vi "WLAN - BCM - PL.vi"(6 "RX ?":bool, 11 "Channel index":i32=1) -> (3 "PL":dbl=17.6)   [LabVIEW 2012]
panel:
  in  "PL_channel Index":dbl[](array[numeric])=[0.0, 17.6, 0.0, 0.0, 0.0, 0.0, 0.0, 17.4, 0.0, 0.0, 0.0, 0.0, 0.0, 17.2, 0.0, 0.0, 0.0, 0.0, 0.0, 0.0, 0.0, 0.0, 0.0, 0.0, 0.0, 0.0, 0.0, 0.0, 0.0, 0.0, 0.0, 0.0, 0.0, 0.0, 0.0, 0.0, 16.5, 0.0, 17.6, 0.0, 0.0, 0.0, 0.0, 0.0, 0.0, 0.0, 17.75, 0.0, 0.0, 0.0, 0.0, 0.0, 16.75, 0.0, 0.0, 0.0, 0.0, 0.0, 0.0, 0.0, 0.0, 0.0, 17.75, 0.0, 16.75, 0.0, 0.0, 0.0, 0.0, 0.0, 0.0, 0.0, 0.0, 0.0, 0.0, 0.0, 0.0, 0.0, 0.0, 0.0, 0.0, 0.0, 0.0, 0.0, 0.0, 0.0, 0.0, 0.0, 0.0, 0.0, 0.0, 0.0, 0.0, 0.0, 0.0, 0.0, 0.0, 0.0, 0.0, 0.0, 16.75, 0.0, 17.9, 0.0, 0.0, 0.0, 0.0, 0.0, 0.0, 0.0, 0.0, 0.0, 0.0, 0.0, 0.0, 0.0, 0.0, 0.0, 0.0, 0.0, 16.75, 0.0, 0.0, 0.0, 0.0, 0.0, 17.9, 0.0, 0.0, 0.0, 0.0, 0.0, 0.0, 0.0, 17.7, 0.0, 0.0, 0.0, 0.0, 0.0, 16.7, 0.0, 0.0, 0.0, 0.0, 0.0, 0.0, 0.0, 0.0, 16.5, 0.0, 17.8, 0.0, 0.0, 0.0, 0.0, 0.0, 16.75, 0.0, 17.9, 0.0, 0.0, 0.0, 0.0, 0.0, 16.75]
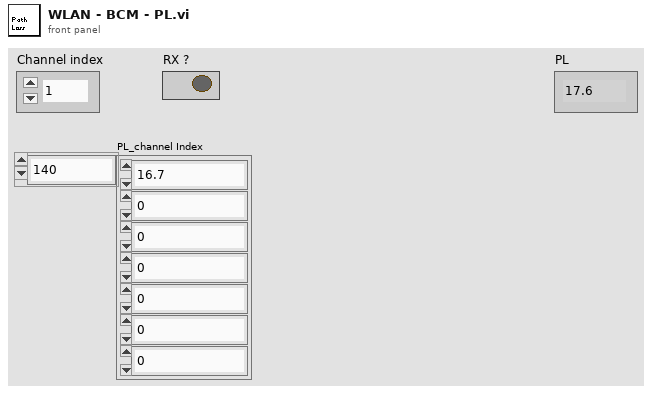
[diagram p1: front panel]
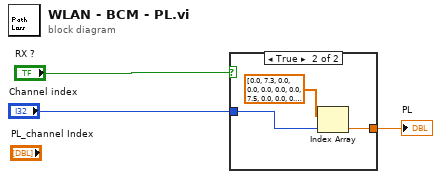
[diagram p0: block diagram]
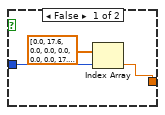
[diagram p2: hidden frame]
diagram:
  n1 = case shown="True" "RX ?" {
    tunnel: [w5 w7] -> w2
    tunnel: "Channel index" -> [w4 w8]
    frame False {
      n2 = Index Array(array=dbl[] [0.0, 17.6, 0.0, 0.0, 0.0, 0.0, 0.0, 17.4, 0.0, 0.0, 0.0, 0.0, 0.0, 17.2, 0.0, 0.0, 0.0, 0.0, 0.0, 0.0, 0.0, 0.0, 0.0, 0.0, 0.0, 0.0, 0.0, 0.0, 0.0, 0.0, 0.0, 0.0, 0.0, 0.0, 0.0, 0.0, 16.5, 0.0, 17.6, 0.0, 0.0, 0.0, 0.0, 0.0, 0.0, 0.0, 17.75, 0.0, 0.0, 0.0, 0.0, 0.0, 16.75, 0.0, 0.0, 0.0, 0.0, 0.0, 0.0, 0.0, 0.0, 0.0, 17.75, 0.0, 16.75, 0.0, 0.0, 0.0, 0.0, 0.0, 0.0, 0.0, 0.0, 0.0, 0.0, 0.0, 0.0, 0.0, 0.0, 0.0, 0.0, 0.0, 0.0, 0.0, 0.0, 0.0, 0.0, 0.0, 0.0, 0.0, 0.0, 0.0, 0.0, 0.0, 0.0, 0.0, 0.0, 0.0, 0.0, 0.0, 16.75, 0.0, 17.9, 0.0, 0.0, 0.0, 0.0, 0.0, 0.0, 0.0, 0.0, 0.0, 0.0, 0.0, 0.0, 0.0, 0.0, 0.0, 0.0, 0.0, 16.75, 0.0, 0.0, 0.0, 0.0, 0.0, 17.9, 0.0, 0.0, 0.0, 0.0, 0.0, 0.0, 0.0, 17.7, 0.0, 0.0, 0.0, 0.0, 0.0, 16.7, 0.0, 0.0, 0.0, 0.0, 0.0, 0.0, 0.0, 0.0, 16.5, 0.0, 17.8, 0.0, 0.0, 0.0, 0.0, 0.0, 16.75, 0.0, 17.9, 0.0, 0.0, 0.0, 0.0, 0.0, 16.75] ("PL_channel Index"), index=w4) -> (element=w5:dbl)
    }
    frame True {
      n3 = Index Array(array=dbl[] [0.0, 7.3, 0.0, 0.0, 0.0, 0.0, 0.0, 7.5, 0.0, 0.0, 0.0, 0.0, 0.0, 7.1, 0.0, 0.0, 0.0, 0.0, 0.0, 0.0, 0.0, 0.0, 0.0, 0.0, 0.0, 0.0, 0.0, 0.0, 0.0, 0.0, 0.0, 0.0, 0.0, 0.0, 0.0, 0.0, 7.8, 0.0, 8.1, 0.0, 0.0, 0.0, 0.0, 0.0, 0.0, 0.0, 8.0, 0.0, 0.0, 0.0, 0.0, 0.0, 8.0, 0.0, 0.0, 0.0, 0.0, 0.0, 0.0, 0.0, 0.0, 0.0, 7.9, 0.0, 8.0, 0.0, 0.0, 0.0, 0.0, 0.0, 0.0, 0.0, 0.0, 0.0, 0.0, 0.0, 0.0, 0.0, 0.0, 0.0, 0.0, 0.0, 0.0, 0.0, 0.0, 0.0, 0.0, 0.0, 0.0, 0.0, 0.0, 0.0, 0.0, 0.0, 0.0, 0.0, 0.0, 0.0, 0.0, 0.0, 8.5, 0.0, 8.5, 0.0, 0.0, 0.0, 0.0, 0.0, 0.0, 0.0, 0.0, 0.0, 0.0, 0.0, 0.0, 0.0, 0.0, 0.0, 0.0, 0.0, 8.3, 0.0, 0.0, 0.0, 0.0, 0.0, 7.9, 0.0, 0.0, 0.0, 0.0, 0.0, 0.0, 0.0, 8.4, 0.0, 0.0, 0.0, 0.0, 0.0, 8.0, 0.0, 0.0, 0.0, 0.0, 0.0, 0.0, 0.0, 0.0, 8.3, 0.0, 8.3, 0.0, 0.0, 0.0, 0.0, 0.0, 8.1, 0.0, 8.0, 0.0, 0.0, 0.0, 0.0, 0.0, 8.2] ("PL_channel Index"), index=w8) -> (element=w7:dbl)
    }
  }
  "PL" <- w2
